vi "数据查询_数据查询.vi"() -> ()   [LabVIEW 2016]
uses:
  <vilib>/Utility/miscctls.llb/LVPointTypeDef.ctl
  <vilib>/Utility/miscctls.llb/LVRowAndColumnUnsignedTypeDef.ctl
  <vilib>/addons/database/_DB Variant To Data/Database Variant To Data.xnode
panel:
  in  "工作模式":string(combo)="全部数据"
  out "连接的字符串":string
  out "选中数据表":string
  in  "查询":bool
  in  "结束日期":string="2020/01/01"
  in  "起始日期":string="2010/01/01"
  out "XY图":cluster{"data":timestamp[], "data":dbl[]}[](graph)
  in  "组合框":string(combo)
  out "数据表":string[][](table)
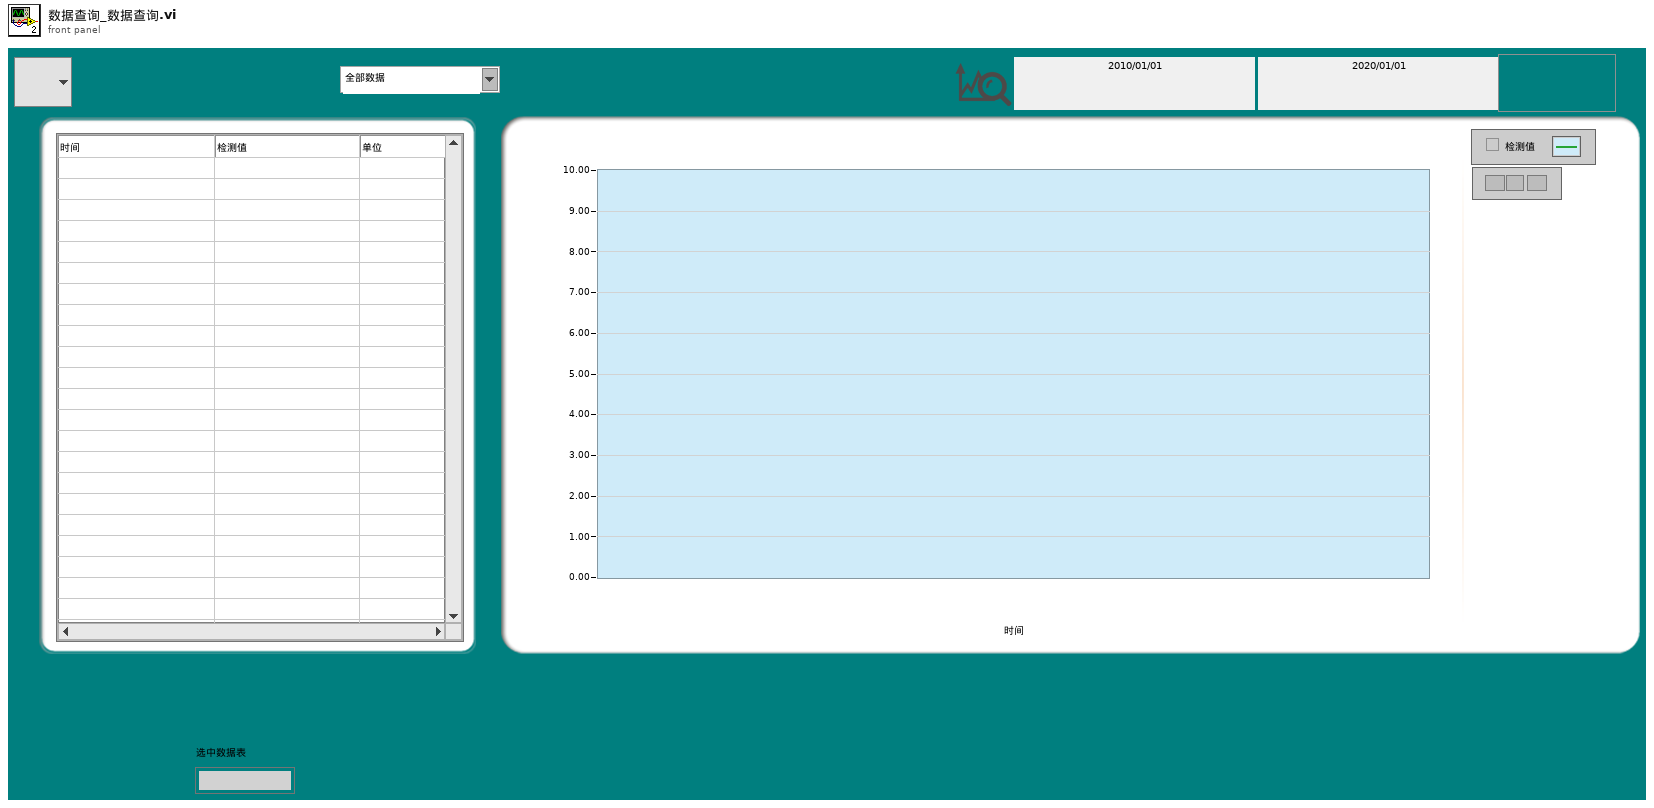
[diagram p1: front panel]
types:
  T1 = typedef "LVPointTypeDef.ctl" = cluster{"Horizontal":i16, "Vertical":i16}
  T2 = typedef "LVRowAndColumnUnsignedTypeDef.ctl" = cluster{"Row":u32, "Column":u32}
  T3 = typedef "LVPoint32TypeDef.ctl" = cluster{"Horizontal":i32, "Vertical":i32}
  T4 = typedef "LVPointDoubleTypeDef.ctl" = cluster{"Cursor X":dbl, "Cursor Y":dbl}
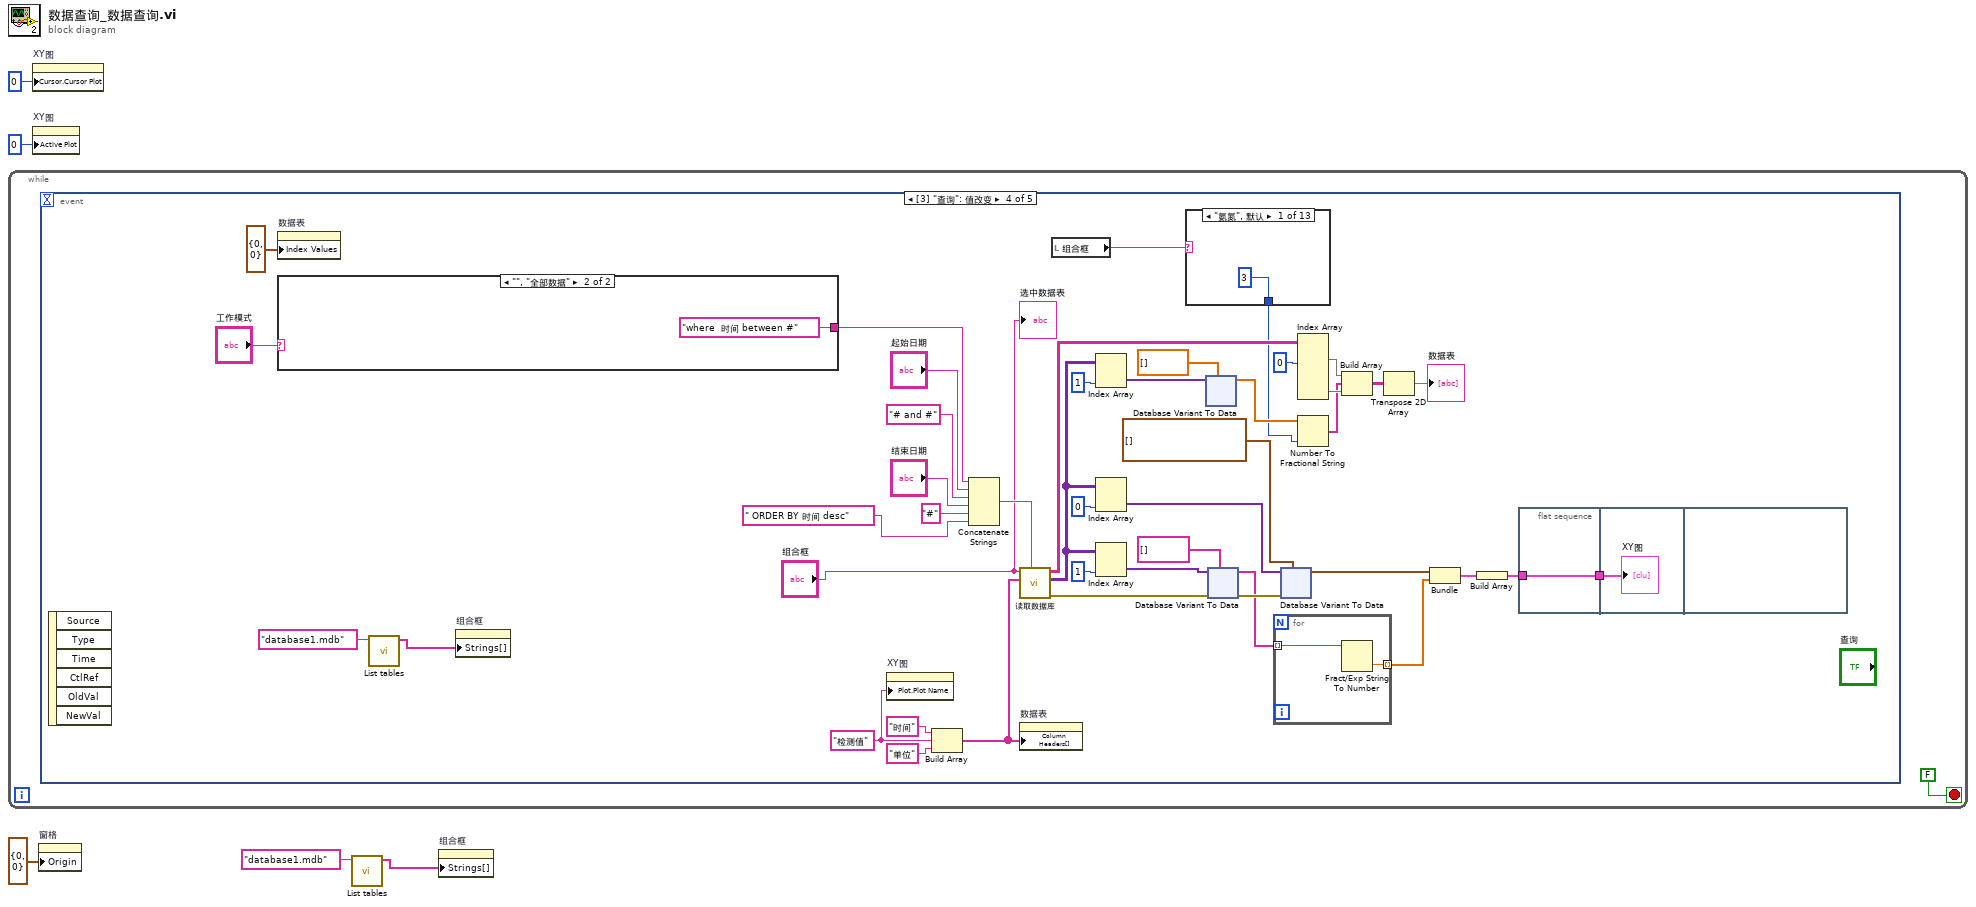
[diagram p0: block diagram]
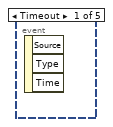
[diagram p2: hidden frame]
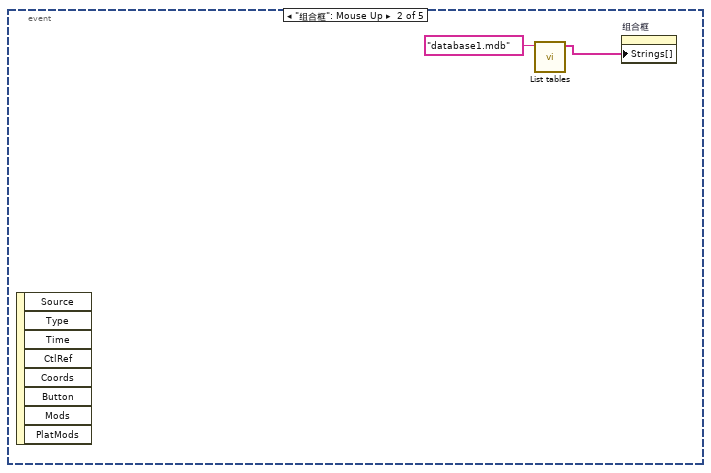
[diagram p3: hidden frame]
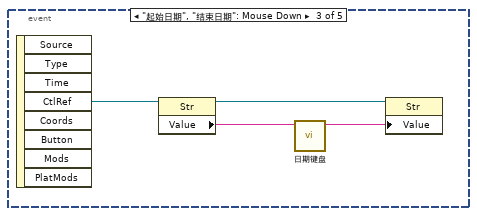
[diagram p4: hidden frame]
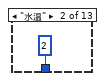
[diagram p5: hidden frame]
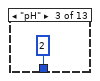
[diagram p6: hidden frame]
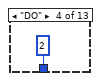
[diagram p7: hidden frame]
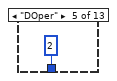
[diagram p8: hidden frame]
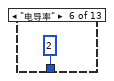
[diagram p9: hidden frame]
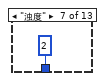
[diagram p10: hidden frame]
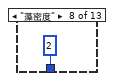
[diagram p11: hidden frame]
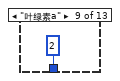
[diagram p12: hidden frame]
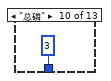
[diagram p13: hidden frame]
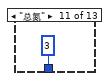
[diagram p14: hidden frame]
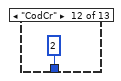
[diagram p15: hidden frame]
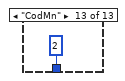
[diagram p16: hidden frame]
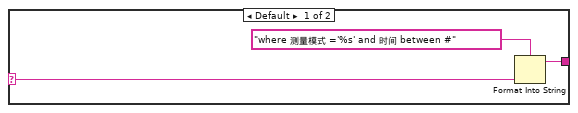
[diagram p17: hidden frame]
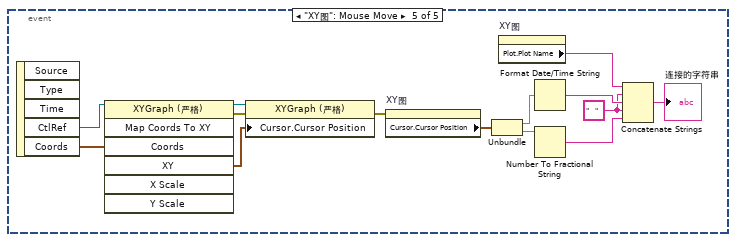
[diagram p18: hidden frame]
diagram:
  n1 = while {
    stop <- FALSE stop-if-true
    n2 = event shown="[3] \"查询\": 值改变" {
      selector: _ -> [_ _ _ _ _]
      dyn-events: _ -> [_ _ _ _ _]
      timeout: _ -> [_ _ _ _ _]
      event Timeout {
        n3 = event-data() -> ()  [unwired: 1 in, 3 out]
      }
      event "组合框": Mouse Up {
        n4 = event-data() -> ()  [unwired: 1 in, 8 out]
        n5 = call "List tables.vi"("database"="database1.mdb") -> ("tables"=w8:string[])  [unwired: 9 in, 1 out]
        n6 = property on="组合框" class="CmbBox"("Strings[]"=w8) -> ()  [unwired: 2 in, 2 out]
      }
      event "起始日期", "结束日期": Mouse Down {
        n7 = event-data() -> ("CtlRef"=w12:refnum<vi>)  [unwired: 1 in, 7 out]
        n8 = property class="Str"(reference=w12) -> (reference out=w10:refnum<vi>, "Value"=w11:string)  [unwired: 1 in, 1 out]
        n9 = call "日期键盘.vi"("原值"=w11) -> ("x+y"=w9:string)  [unwired: 10 in]
        n10 = property class="Str"(reference=w10, "Value"=w9) -> ()  [unwired: 1 in, 2 out]
      }
      event "查询": Value Change {
        w30 = "检测值"
        n11 = event-data() -> ()  [unwired: 1 in, 6 out]
        n12 = property on="数据表" class="Tbl (严格)"("Index Values"=T2 {"Row"=0, "Column"=0} ("索引值")) -> ()  [unwired: 2 in, 2 out]
        n13 = case shown="\"\", \"全部数据\"" "工作模式" {
          selector: "工作模式" -> [w72 _]
          tunnel: [w70 "where  时间 between #" ("condition")] -> w19
          frame Default {
            n14 = Format Into String(format string="where 测量模式 ='%s' and 时间 between #" ("condition"), w72) -> (resulting string=w70:string)  [unwired: 2 in, 1 out]
          }
          frame "", "全部数据" {
          }
        }
        n15 = call "List tables.vi"("database"="database1.mdb") -> ("tables"=w14:string[])  [unwired: 9 in, 1 out]
        n16 = property on="组合框" class="CmbBox"("Strings[]"=w14) -> ()  [unwired: 2 in, 2 out]
        n17 = property on="XY图" class="XYGraph (严格)"("Plot.Plot Name"=w30) -> ()  [unwired: 2 in, 2 out]
        n18 = Build Array("时间", w30, "单位" ("元素")) -> (w32:string[])
        n19 = Concatenate Strings(w19, "起始日期", "# and #" ("condition"), "结束日期", "#" ("condition"), " ORDER BY 时间 desc" ("字符串")) -> (w55:string)
        n20 = call "读取数据库.vi"("condition"=w55, "显示项"=w32, "组合框"="组合框") -> ("error out"=w46:errorcluster, "data"=w27:variant[][], "表格"=w38:string[][])  [unwired: 5 in, 1 out]
        n21 = property on="数据表" class="Tbl (严格)"("Column Headers[]"=w32) -> ()  [unwired: 2 in, 2 out]
        n22 = local read "组合框"() -> (w17:string)
        n23 = Index Array(array=w27, index (col)=1 ("禁用的索引 (列)")) -> (element=w25:variant[])  [unwired: 1 in]
        n24 = Index Array(array=w27, index (col)=0 ("禁用的索引 (列)")) -> (element=w49:variant[])  [unwired: 1 in]
        n25 = Index Array(array=w27, index (col)=1 ("禁用的索引 (列)")) -> (element=w47:variant[])  [unwired: 1 in]
        n26 = case shown="\"氨氮\", 默认" w17 {
          tunnel: [i16 3 ("精度(6)") i16 2 ("精度(6)") i16 2 ("精度(6)") i16 2 ("精度(6)") i16 2 ("精度(6)") i16 2 ("精度(6)") i16 2 ("精度(6)") i16 2 ("精度(6)") i16 2 ("精度(6)") i16 3 ("精度(6)") i16 3 ("精度(6)") i16 2 ("精度(6)") i16 2 ("精度(6)")] -> w16
          frame "氨氮", Default {
          }
          frame "水温" {
          }
          frame "pH" {
          }
          frame "DO" {
          }
          frame "DOper" {
          }
          frame "电导率" {
          }
          frame "浊度" {
          }
          frame "藻密度" {
          }
          frame "叶绿素a" {
          }
          frame "总磷" {
          }
          frame "总氮" {
          }
          frame "CodCr" {
          }
          frame "CodMn" {
          }
        }
        n27 = xnode "Database Variant To Data"("database variant"=w25, "type"=sgl[] []) -> ("data"=w23:sgl[])  [unwired: 1 in, 1 out]
        n28 = xnode "Database Variant To Data"("database variant"=w47, "error in (no error)"=w46, "type"=string[] []) -> ("data"=w31:string[], "error out"=w45:errorcluster)
        n29 = for {
          tunnel: w31 -> [w113] mode=indexing
          tunnel: [w112] -> w18 mode=indexing
          n30 = Fract/Exp String To Number(string=w113) -> (number=w112:dbl)  [unwired: 3 in, 1 out]
        }
        n31 = xnode "Database Variant To Data"("database variant"=w49, "error in (no error)"=w45, "type"=timestamp[] []) -> ("data"=w40:timestamp[])  [unwired: 1 out]
        n32 = Index Array(array=w38, index (col) #1=0 ("禁用的索引 (列)")) -> (element #1=w36:string[], element #3=w28:string[])  [unwired: 5 in, 1 out]
        n33 = Number To Fractional String(number=w23, precision (6)=w16) -> (F-format string=w22:string[])  [unwired: 2 in]
        n34 = Build Array(w36, w22, w28) -> (w35:string[][])
        n35 = Transpose 2D Array(2D array=w35) -> (transposed array=→"数据表":string[][])
        n36 = Bundle("data"=w40, w18) -> (w41:cluster{"data":timestamp[], dbl[]})  [unwired: 1 in]
        n37 = Build Array(w41) -> (w42:cluster{"data":timestamp[], dbl[]}[])
        n38 = flat-sequence {
          tunnel: [w114] -> w43
          tunnel: w42 -> [w114]
          tunnel: w43 -> [w115]
          frame #0 {
          }
          frame #1 {
            "XY图" <- w115
          }
          frame #2 {
          }
        }
        "选中数据表" <- "组合框"
      }
      event "XY图": Mouse Move {
        w209 = "   " ("字符串")
        n39 = event-data() -> ("CtlRef"=w219:refnum<vi>, "Coords"=w218:T3)  [unwired: 1 in, 3 out]
        n40 = invoke class="XYGraph (严格)" method="Map Coords To XY"(reference=w219, "Coords"=w218) -> (reference out=w217:refnum<vi>, error out=w214:errorcluster, "XY"=w216:cluster{"X":dbl, "Y":dbl})  [unwired: 5 in, 4 out]
        n41 = property class="XYGraph (严格)"(reference=w217, error in=w214, "Cursor.Cursor Position"=w216) -> (error out=w215:errorcluster)  [unwired: 1 out]
        n42 = property on="XY图" class="XYGraph (严格)"(error in=w215) -> ("Cursor.Cursor Position"=w212:T4)  [unwired: 1 in, 2 out]
        n43 = Unbundle(w212) -> ("Cursor X"=w211:dbl, "Cursor Y"=w208:dbl)
        n44 = property on="XY图" class="XYGraph (严格)"() -> ("Plot.Plot Name"=w206:string)  [unwired: 2 in, 2 out]
        n45 = Format Date/Time String(seconds (now)=w211) -> (date/time string=w210:string)  [unwired: 2 in]
        n46 = Number To Fractional String(number=w208) -> (F-format string=w207:string)  [unwired: 3 in]
        n47 = Concatenate Strings(w206, w209, w210, w209, w207) -> (→"连接的字符串":string)
      }
    }
  }
  n48 = property on="XY图" class="XYGraph (严格)"("Cursor.Cursor Plot"=0 ("游标.游标关联曲线")) -> ()  [unwired: 2 in, 2 out]
  n49 = property on="XY图" class="XYGraph (严格)"("Active Plot"=u32 0 ("活动曲线")) -> ()  [unwired: 2 in, 2 out]
  n50 = property on="窗格" class="Pane"("Origin"=T1 {"Horizontal"=0, "Vertical"=0} ("原点")) -> ()  [unwired: 2 in, 2 out]
  n51 = call "List tables.vi"("database"="database1.mdb") -> ("tables"=w1:string[])  [unwired: 9 in, 1 out]
  n52 = property on="组合框" class="CmbBox"("Strings[]"=w1) -> ()  [unwired: 2 in, 2 out]
